vi "_Edit Labels GUI.vi"(0 "labels in":string[](array[string])) -> (4 "labels out":string[](array[string]), 6 "canceled":bool)   [LabVIEW 2015]
uses:
  <vilib>/Analysis/baseanly.llb/Mean (DBL).vi
  <userlib>/LV System Utils v1/LV System Utils v1.lvlib
  <userlib>/LV String Utils v1/LV String Utils v1.lvlib
  <vilib>/Analysis/NI_AALBase.lvlib
panel:
  in  "Tab Control":enum32{"Preview", "Code", "Error"}(tab)=enum."Code"
  in  "Cancel":bool
  in  "OK":bool
  in  "Preview":string[][](array[string])
  in  "Code":string="for label in labels:\n    print(label)\n"
  in  "Execute":bool
  in  "Scripts":string(combo)="<default>"
  in  "Error":string
  # "Old values"
  # "New values"
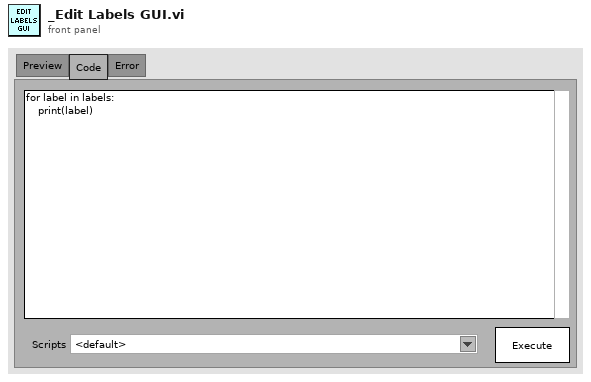
[diagram p1: front panel]
types:
  T1 = typedef "LVPoint32TypeDef.ctl" = cluster{"Horizontal":i32, "Vertical":i32}
  T2 = typedef "LVRectTypeDef.ctl" = cluster{"Left":i16, "Top":i16, "Right":i16, "Bottom":i16}
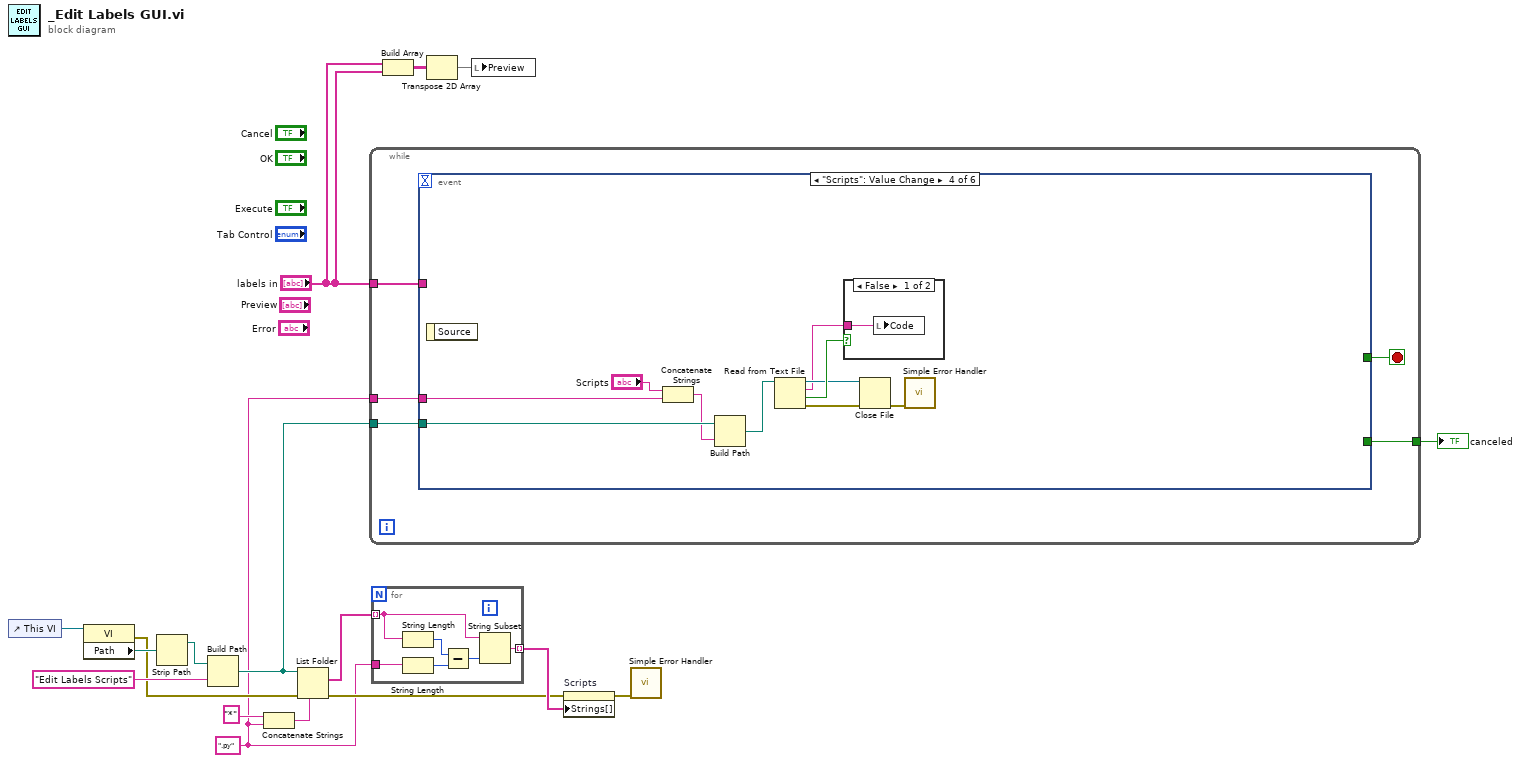
[diagram p0: block diagram]
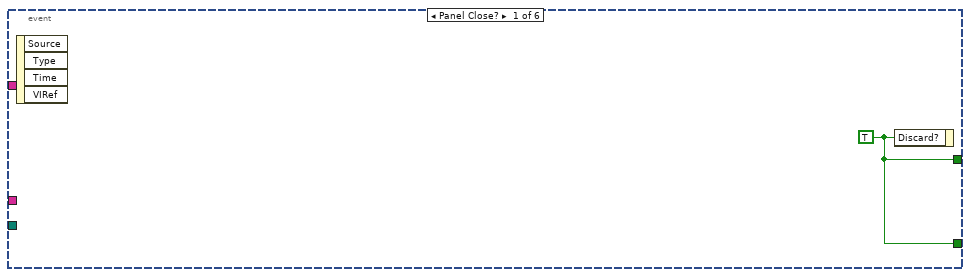
[diagram p2: hidden frame]
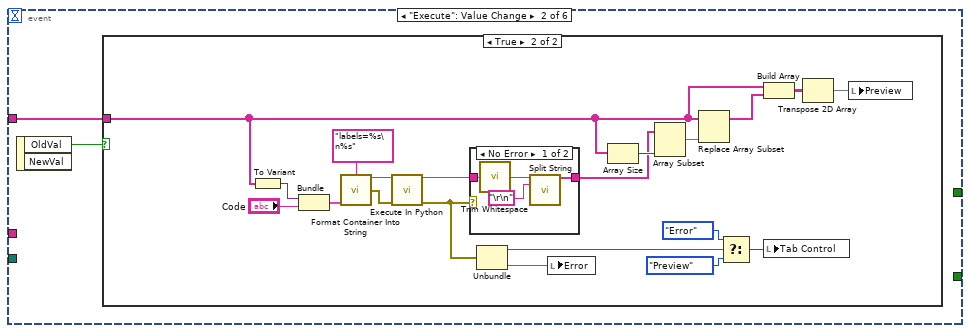
[diagram p3: hidden frame]
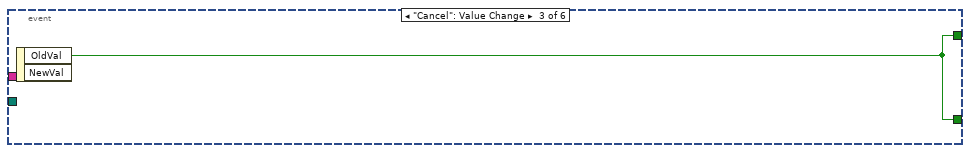
[diagram p6: hidden frame]
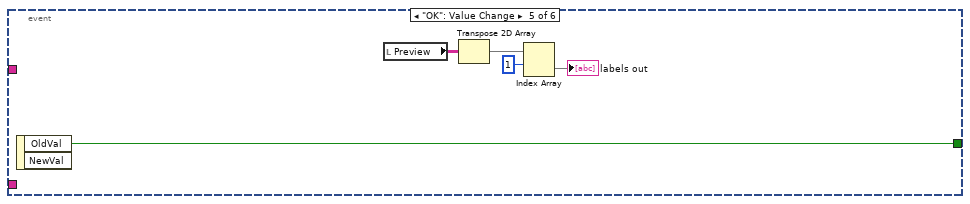
[diagram p8: hidden frame]
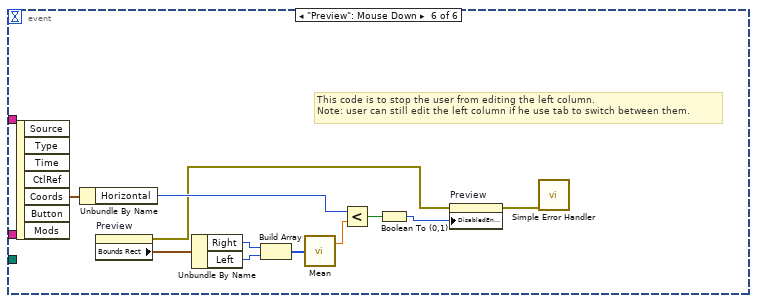
[diagram p9: hidden frame]
diagram:
  w1 = ".py" ("pattern")
  n1 = control-ref of="This VI"() -> (w13:refnum<vi>)
  n2 = property class="VI"(reference=w13) -> (error out=w7:errorcluster, "Path"=w12:path)  [unwired: 1 in, 1 out]
  n3 = Strip Path(path=w12) -> (stripped path=w11:path)  [unwired: 1 out]
  n4 = Build Path(base path=w11, name or relative path="Edit Labels Scripts") -> (appended path=w2:path)
  n5 = Concatenate Strings("*" ("pattern"), w1) -> (w3:string)
  n6 = List Folder(path=w2, pattern=w3, error in=w7) -> (filenames=w5:string[], error out=w6:errorcluster)  [unwired: 1 in, 2 out]
  n7 = while {
    tunnel: "labels in" -> [w21]
    tunnel: [w20] -> w17
    tunnel: w2 -> [w19]
    tunnel: w1 -> [w18]
    stop <- w22 stop-if-true
    n8 = event shown="[3] \"Scripts\": Value Change" {
      selector: _ -> [_ _ _ _ _ _]
      dyn-events: _ -> [_ _ _ _ _ _]
      timeout: _ -> [_ _ _ _ _ _]
      tunnel: [w23 _ w50 _ w66 _] -> w22
      tunnel: w21 -> [_ w24 _ _ _ _]
      tunnel: [w23 _ w50 _ _ _] -> w20
      tunnel: w19 -> [_ _ _ w60 _ _]
      tunnel: w18 -> [_ _ _ w59 _ _]
      event Panel Close? {
        w23 = TRUE ("Discard?")
        n9 = event-data() -> ()  [unwired: 1 in, 4 out]
        n10 = event-data("Discard?"=w23) -> ()  [unwired: 1 in, 1 out]
      }
      event "Execute": Value Change {
        n11 = event-data() -> ("OldVal"=w25:bool)  [unwired: 1 in, 1 out]
        n12 = case shown="True" w25 {
          tunnel: w24 -> [_ w30]
          frame False {
          }
          frame True {
            n13 = To Variant(anything=w30) -> (Variant=w39:variant)
            n14 = Bundle("Variant"=w39, "Code"="Code") -> (w38:cluster{"Variant":variant, "Code":string})  [unwired: 1 in]
            n15 = call <userlib>:"Format Container Into String.vi"("format string"="labels=%s\n%s", "input"=w38) -> ("resulting string"=w40:string, "error out"=w36:errorcluster)  [unwired: 12 in]
            n16 = call <userlib>:"Execute In Python.vi"("code"=w40, "error in (no error)"=w36) -> ("stdout"=w43:string, "error out"=w45:errorcluster)  [unwired: 12 in]
            n17 = case shown="No Error" w45 {
              tunnel: [w48 _] -> w41
              tunnel: w43 -> [w47 _]
              frame No Error {
                n18 = call <vilib>:"Trim Whitespace.vi"("string"=w47) -> ("trimmed string"=w46:string)  [unwired: 1 in]
                n19 = call <userlib>:"Split String.vi"("string in"=w46, "separator"="\r\n") -> ("string array"=w48:string[])  [unwired: 13 in]
              }
              frame Error {
              }
            }
            n20 = Unbundle(w45) -> ("status"=w34:bool, "source"=w26:string)  [unwired: 1 out]
            n21 = local write "Error"(w26) -> ()
            n22 = Array Size(array=w30) -> (size(s)=w42:i32)
            n23 = Array Subset(array=w41, length=w42) -> (w44:string[])  [unwired: 1 in]
            n24 = Replace Array Subset(array=w30, new element=w44) -> (w29:string[])  [unwired: 1 in]
            n25 = Select(t=enum32{"Preview", "Code", "Error"}."Error" ("Tab Control"), s=w34, f=enum32{"Preview", "Code", "Error"}."Preview" ("Tab Control")) -> (s? t:f=w31:enum32{"Preview", "Code", "Error"})
            n26 = Build Array(w30, w29) -> (w28:string[][])
            n27 = local write "Tab Control"(w31) -> ()
            n28 = Transpose 2D Array(2D array=w28) -> (transposed array=w27:string[][])
            n29 = local write "Preview"(w27) -> ()
          }
        }
      }
      event "Cancel": Value Change {
        n30 = event-data() -> ("OldVal"=w50:bool)  [unwired: 1 in, 1 out]
      }
      event "Scripts": Value Change {
        n31 = event-data() -> ()  [unwired: 1 in, 1 out]
        n32 = Concatenate Strings("Scripts", w59) -> (w57:string)
        n33 = Build Path(base path=w60, name or relative path=w57) -> (appended path=w56:path)
        n34 = Read from Text File(file (use dialog)=w56) -> (refnum out=w52:refnum<file>, text=w51:string, cancelled=w55:bool, error out=w54:errorcluster)  [unwired: 3 in]
        n35 = case shown="False" w55 {
          tunnel: w51 -> [w61 _]
          frame False {
            n36 = local write "Code"(w61) -> ()
          }
          frame True {
          }
        }
        n37 = Close File(refnum=w52, error in=w54) -> (error out=w53:errorcluster)  [unwired: 1 out]
        n38 = call <vilib>:"Simple Error Handler.vi"("error in (no error)"=w53) -> ()  [unwired: 4 in, 5 out]
      }
      event "OK": Value Change {
        n39 = event-data() -> ("OldVal"=w66:bool)  [unwired: 1 in, 1 out]
        n40 = local read "Preview"() -> (w62:string[][])
        n41 = Transpose 2D Array(2D array=w62) -> (transposed array=w65:string[][])
        n42 = Index Array(array=w65, index (row)=1 ("disabled index (col)")) -> (element=→"labels out":string[])  [unwired: 1 in]
      }
      event "Preview": Mouse Down {
        # "This code is to stop the user from editing the left column.\nNote: user can still edit the left column if he use tab to switch between them."
        n43 = event-data() -> ("Coords"=w77:T1)  [unwired: 1 in, 6 out]
        n44 = Unbundle By Name(w77) -> ("Horizontal"=w75:i32)
        n45 = property on="Preview" class="Arr (strict)"() -> (error out=w68:errorcluster, "Bounds Rect"=w76:T2)  [unwired: 2 in, 1 out]
        n46 = Unbundle By Name(w76) -> ("Right"=w73:i16, "Left"=w74:i16)
        n47 = Build Array(w73, w74) -> (w72:i16[])
        n48 = call-poly <vilib>:"Mean.vi"("X"=w72) -> ("mean"=w71:dbl)  [unwired: 1 out]
        n49 = Less?(x=w75, y=w71) -> (x < y?=w70:bool)
        n50 = Boolean To (0,1)(Boolean=w70) -> (0, 1=w69:i16)
        n51 = property on="Preview" class="Arr (strict)"(error in=w68, "DisabledEnum"=w69) -> (error out=w67:errorcluster)  [unwired: 1 in, 1 out]
        n52 = call <vilib>:"Simple Error Handler.vi"("error in (no error)"=w67) -> ()  [unwired: 4 in, 5 out]
      }
    }
  }
  "canceled" <- w17
  n53 = for {
    tunnel: w5 -> [w81] mode=indexing
    tunnel: [w80] -> w8 mode=indexing
    tunnel: w1 -> [w78]
    n54 = String Length(string=w81) -> (length=w83:i32)
    n55 = String Length(string=w78) -> (length=w79:i32)
    n56 = Subtract(x=w83, y=w79) -> (x-y=w82:i32)
    n57 = String Subset(string=w81, length (rest)=w82) -> (substring=w80:string)  [unwired: 1 in]
  }
  n58 = Build Array("labels in", "labels in") -> (w15:string[][])
  n59 = Transpose 2D Array(2D array=w15) -> (transposed array=w14:string[][])
  n60 = local write "Preview"(w14) -> ()
  n61 = property on="Scripts" class="CmbBox"(error in=w6, "Strings[]"=w8) -> (error out=w9:errorcluster)  [unwired: 1 in, 1 out]
  n62 = call <vilib>:"Simple Error Handler.vi"("error in (no error)"=w9) -> ()  [unwired: 4 in, 5 out]
